vi "SMBUS Block Write.vi"(4 "WithPEC":u8, 5 "WriteCount":i32, 6 "pWriteData":u8, 7 "CommandCode":u8, 9 "SlaveAddr":i16, 10 "IICIndex":i32, 11 "DevHandle":i32) -> (2 "function return":i32, 3 "pWriteData out":u8)   [LabVIEW 2010, in "usb2iic.lvlib"]
doc: "int WINAPI SMBUS_BlockWrite(int DevHandle,int IICIndex,short SlaveAddr,unsigned char CommandCode, unsigned char *pWriteData,int WriteCount,unsigned char WithPEC);"
uses:
  usb2iic.lvlib
  USB2XXX.dll
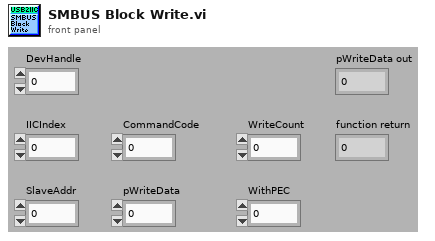
[diagram p1: front panel]
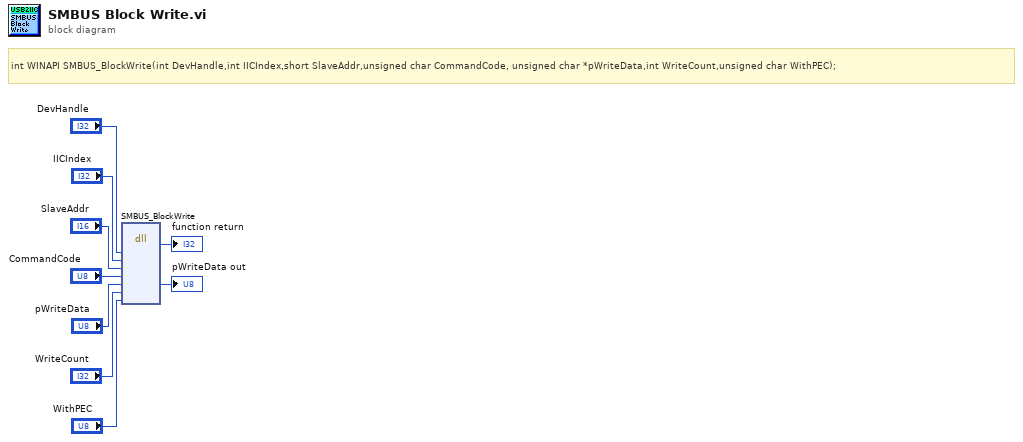
[diagram p0: block diagram]
diagram:
  # "int WINAPI SMBUS_BlockWrite(int DevHandle,int IICIndex,short SlaveAddr,unsigned char CommandCode, unsigned char *pWriteData,int WriteCount,unsigned char WithPEC);"
  n1 = dll-call lib="G:/OtherWork/USB2XXX_Example/trunk/Labview/PublicFiles/usb2iic/USB2XXX.*" fn="SMBUS_BlockWrite"("DevHandle"="DevHandle", "IICIndex"="IICIndex", "SlaveAddr"="SlaveAddr", "CommandCode"="CommandCode", "pWriteData"="pWriteData", "WriteCount"="WriteCount", "WithPEC"="WithPEC") -> (→"function return":i32, "pWriteData"=→"pWriteData out":u8)  [unwired: 9 in, 2 out]
